vi "Read Sdettings.vi"(0 "class data in":refnum<class "MB_ENGINE.lvclass">, 11 "error in (no error)":errorcluster) -> (4 "class data out":refnum<class "MB_ENGINE.lvclass">, 6 "cluster":T1, 15 "error out":errorcluster)   [LabVIEW 2019, in "MB_ENGINE.lvclass"]
uses:
  MB_ENGINE.lvclass
  Settings.ctl
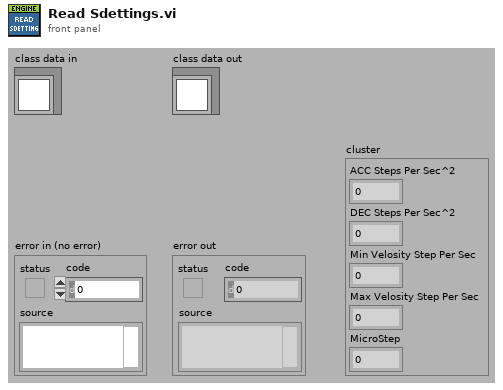
[diagram p1: front panel]
types:
  T1 = typedef "MB_ENGINE.lvclass/Settings.ctl" = cluster{"ACC Steps Per Sec^2":u16, "DEC Steps Per Sec^2":u16, "Min Velosity Step Per Sec":u16, "Max Velosity Step Per Sec":u16, "MicroStep":u16}
  T2 = cluster{"[0]":u16, "[1]":u16, "[2]":u16, "[3]":u16, "[4]":u16}
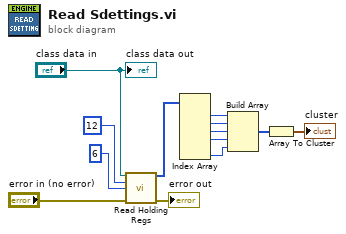
[diagram p0: block diagram]
diagram:
  n1 = call-dynamic "Read Holding Regs.vi"("reference in"="class data in", "starting address"=u16 12, "number of inputs"=u16 6, "error in (no error)"="error in (no error)") -> ("register values"=w7:u16[], "error out"=→"error out":errorcluster)  [unwired: 10 in]
  n2 = Index Array(array=w7) -> (element #1=w5:u16, element #2=w6:u16, element #3=w3:u16, element #4=w2:u16, element #6=w1:u16)  [unwired: 6 in, 1 out]
  n3 = Build Array(w5, w6, w3, w2, w1) -> (w4:u16[])
  n4 = Array To Cluster(array=w4) -> (cluster=→"cluster":T2)
  "class data out" <- "class data in"
